vi "Agilent VNA Measure.vi"(5 "Miscellaneous Parameters":T1, 7 "Agilent VNA":T5, 8 "error in (no error)":errorcluster, 9 "SP Stimulus":T2={"Use Instrument Settings"=FALSE, "Blank Frequencies"=FALSE, "Sweep Type"=enum."Linear", "Sweep"={"Fstart"=500.0, "Fstop"=1500.0, "Units"=enum."MHz", "Points"=201}, "Power (dBm)"=999.0, "IFBW (Hz)"=-1.0, "Sweep Time (s)"=-1.0, "Calibration"={"State"=FALSE, "String"=""}} {"Sweep Time (s)" format="%.3g"}, 10 "Parameters to Measure":T6[](array[typedef]) {"Channel" min=1 max=99 step=1; "Parameter"."Stimulus Port" min=1 step=1; "Parameter"."Response Port" min=1 step=1}, 11 "VISA Resource Name":refnum<visa-resource-name>) -> (0 "error out":errorcluster, 1 "S Parameters":cluster{"f0":dbl, "df":dbl, cdb[][]}, 2 "Parameters to Measure":T6[](array[typedef]) {"Channel" min=1 max=99 step=1; "Parameter"."Stimulus Port" min=1 step=1; "Parameter"."Response Port" min=1 step=1}, 3 "dup VISA Resource Name":refnum<visa-resource-name>)   [LabVIEW 2011]
uses:
  tests/S Parameter/TypeDefs/SP Parameter to Measure.ctl
  tests/S Parameter/TypeDefs/SP Parameter.ctl
  tests/S Parameter/TypeDefs/SP Calibration State.ctl
  tests/S Parameter/TypeDefs/SP Measurement Format.ctl
  TypeDefs/Agilent VNA Instrument Info.ctl
  tests/S Parameter/TypeDefs/SP Stimulus Parameters.ctl
  tests/S Parameter/TypeDefs/SP Frequency Units.ctl
  tests/S Parameter/TypeDefs/SP Miscellaneous Parameters.ctl
  TypeDefs/Agilent VNA External Trigger Mode.ctl
  TypeDefs/Agilent VNA Measurement.ctl
  TypeDefs/Agilent VNA Trigger Mode.ctl
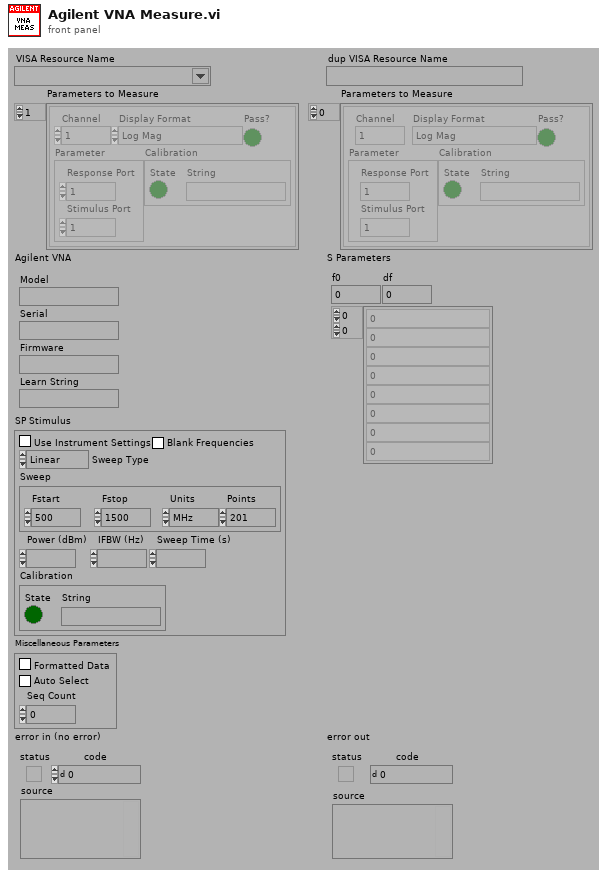
[diagram p1: front panel]
types:
  T1 = typedef "SP Miscellaneous Parameters.ctl" = cluster{"Formatted Data":bool, "Auto Select":bool, "Seq Count":u32}
  T2 = typedef "SP Stimulus Parameters.ctl" = cluster{"Use Instrument Settings":bool, "Blank Frequencies":bool, "Sweep Type":enum32{"Linear", "Logarithmic", "List", "Power", "CW"}, "Sweep":cluster{"Fstart":dbl, "Fstop":dbl, "Units":T3, "Points":i32}, "Power (dBm)":dbl, "IFBW (Hz)":dbl, "Sweep Time (s)":dbl, "Calibration":T4}
  T3 = typedef "SP Frequency Units.ctl" = enum16{"Hz", "kHz", "MHz", "GHz", "Points"}
  T4 = typedef "SP Calibration State.ctl" = cluster{"State":bool, "String":string}
  T5 = typedef "Agilent VNA Instrument Info.ctl" = cluster{"Model":string, "Serial":string, "Firmware":string, "Learn String":string}
  T6 = typedef "SP Parameter to Measure.ctl" = cluster{"Channel":i8, "Parameter":T7, "Calibration":T4, "Display Format":T8, "Pass?":bool}
  T7 = typedef "SP Parameter.ctl" = cluster{"Stimulus Port":i8, "Response Port":i8}
  T8 = typedef "SP Measurement Format.ctl" = enum32{"Log Mag", "Phase", "Delay", "Smith (R+jX)", "Polar (Re/Im)", "Linear Mag", "SWR", "Real", "Imaginary", "Smith (Lin/Phase)", "Smith (Log/Phase)", "Smith (Real/Imag)", "Smith (G+jB)", "Polar (Lin/Phase)", "Polar (Log/Phase)", "Expanded Phase", "Positive Phase", "Inverted Smith", "Unwrapped Phase", "Power Out", "Power In", "Linear Mag/Phase", "Log Mag/Phase", "Real/Imaginary"}
  T9 = typedef "Agilent VNA Model.ctl" = enum16{"Not Supported", "8510X", "8719X", "8720X", "8722X", "8753X", "ENA", "PNA", "Field Fox"}
  T10 = typedef "Agilent VNA Measurements.ctl" = cluster{"Channel":i8, "Traces":cluster{"Trace":i8, "Parameter":T7}[]}
  T11 = typedef "Agilent VNA External Trigger Mode.ctl" = enum16{"Off", "On Sweep", "On Point", "Manual On Point", "Internal", "External", "Bus"}
  T12 = typedef "Agilent VNA Measurement.ctl" = enum32{"SXX", "Analog In - Aux In", "A/R", "B/R", "A/B", "A", "B", "R"}
  T13 = typedef "Agilent VNA Trigger Mode.ctl" = enum16{"Continuous", "Hold", "Single"}
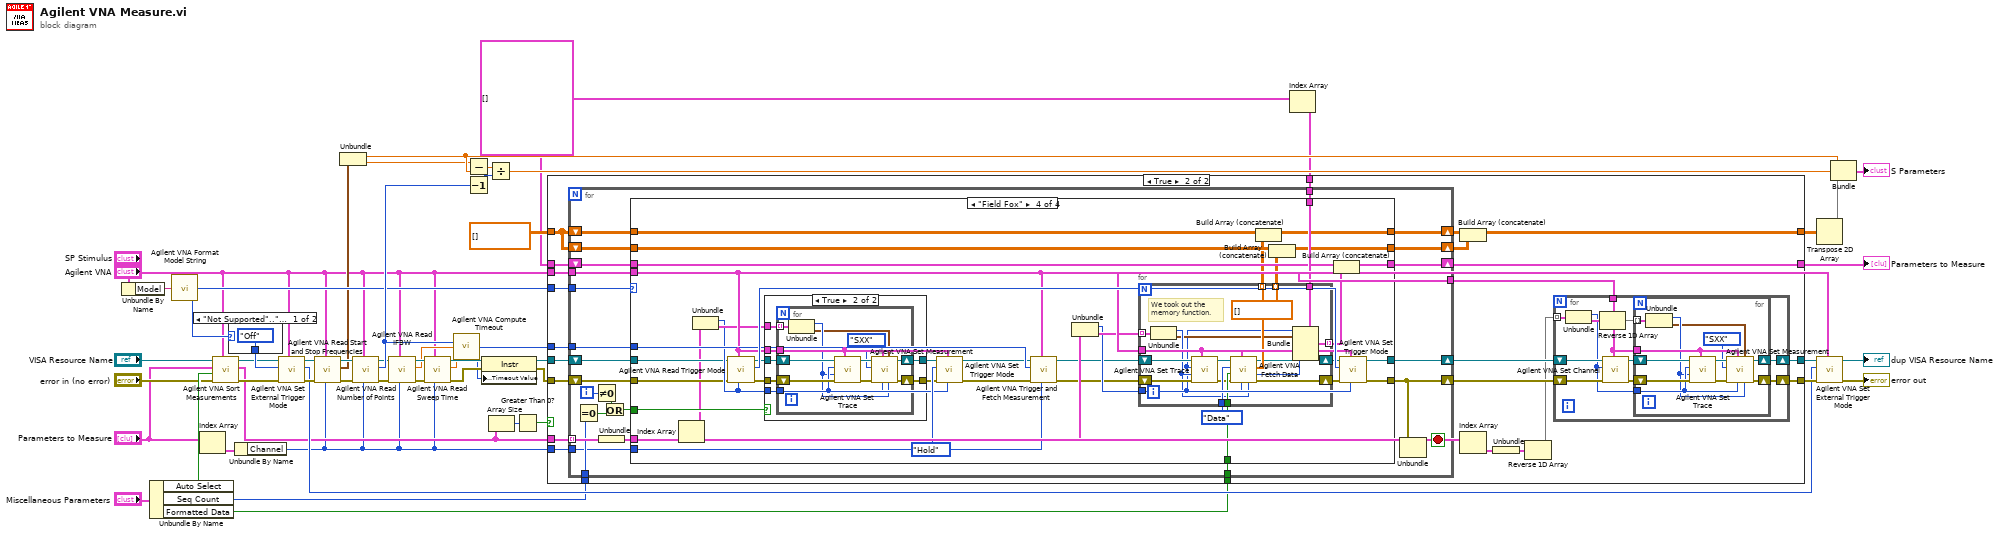
[diagram p0: block diagram]
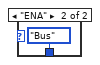
[diagram p2: hidden frame]
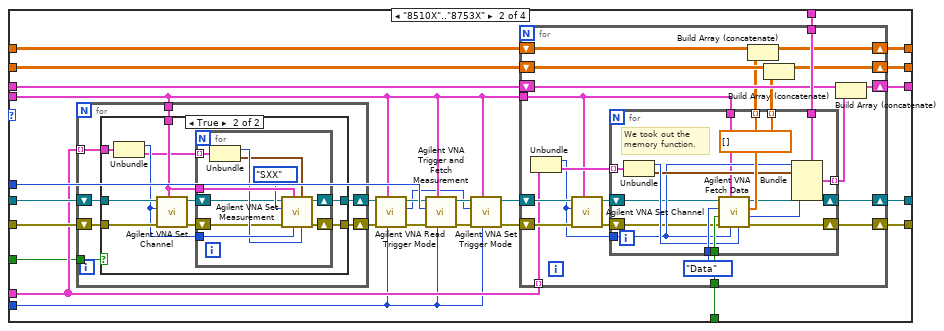
[diagram p5: hidden frame]
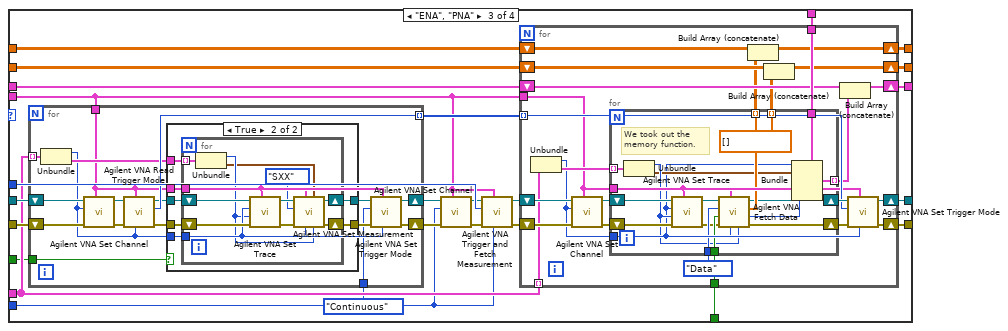
[diagram p7: hidden frame]
diagram:
  w17 = T6[] [] ("Parameters to Measure")
  n1 = Unbundle By Name("Agilent VNA") -> ("Model"=w15:string)
  n2 = Unbundle By Name("Miscellaneous Parameters") -> ("Auto Select"=w9:bool, "Seq Count"=w11:u32, "Formatted Data"=w12:bool)
  n3 = call "Agilent VNA Format Model String.vi"("Model"=w15) -> ("Model"=w14:T9)
  n4 = Index Array(array="Parameters to Measure") -> (element=w3:T6)  [unwired: 1 in]
  n5 = call "Agilent VNA Sort Measurements.vi"("Agilent VNA"="Agilent VNA", "error in (no error)"="error in (no error)", "Auto Select"=w9, "Parameters to Measure"="Parameters to Measure", "VISA Resource Name"="VISA Resource Name") -> ("error out"=w6:errorcluster, "Sorted Measurements"=w4:cluster{"Measurements":T10[]}[], "dup VISA Resource Name"=w7:refnum<visa-resource-name>)  [unwired: 4 out]
  n6 = case shown="\"Not Supported\"..\"8753X\", \"PNA\", \"Field Fox\"" w14 {
    tunnel: [Agilent_VNA_External_Trigger_Mode."Off" ("Ext. Trigger Mode") Agilent_VNA_External_Trigger_Mode."Bus" ("Ext. Trigger Mode")] -> w37
    frame "Not Supported".."8753X", "PNA", "Field Fox" {
    }
    frame "ENA" {
    }
  }
  n7 = Unbundle By Name(w3) -> ("Channel"=w1:i8)
  n8 = call "Agilent VNA Set External Trigger Mode.vi"("Agilent VNA"="Agilent VNA", "error in (no error)"=w6, "Ext. Trigger Mode"=w37, "VISA Resource Name"=w7) -> ("error out"=w26:errorcluster, "Previous Ext. Trigger Mode"=w19:T11, "dup VISA Resource Name"=w25:refnum<visa-resource-name>)  [unwired: 5 out]
  n9 = call "Agilent VNA Read Start and Stop Frequencies.vi"("Channel"=w1, "Agilent VNA"="Agilent VNA", "error in (no error)"=w26, "VISA Resource Name"=w25) -> ("error out"=w21:errorcluster, "Start/Stop Freqs, MHz"=w13:cluster{"Fstart":dbl, "Fstop":dbl}, "dup VISA Resource Name"=w20:refnum<visa-resource-name>)  [unwired: 5 out]
  n10 = Unbundle(w13) -> ("Fstart"=w43:dbl, "Fstop"=w42:dbl)
  n11 = call "Agilent VNA Read Number of Points.vi"("Channel"=w1, "Agilent VNA"="Agilent VNA", "error in (no error)"=w21, "VISA Resource Name"=w20) -> ("error out"=w23:errorcluster, "Number Points"=w27:i32, "dup VISA Resource Name"=w24:refnum<visa-resource-name>)  [unwired: 5 out]
  n12 = call "Agilent VNA Read IFBW.vi"("Channel"=w1, "Agilent VNA"="Agilent VNA", "error in (no error)"=w23, "VISA Resource Name"=w24) -> ("error out"=w35:errorcluster, "IFBW, Hz"=w32:dbl, "dup VISA Resource Name"=w36:refnum<visa-resource-name>)  [unwired: 5 out]
  n13 = call "Agilent VNA Read Sweep Time.vi"("Channel"=w1, "Agilent VNA"="Agilent VNA", "error in (no error)"=w35, "VISA Resource Name"=w36) -> ("error out"=w34:errorcluster, "Sweep Time, s"=w31:dbl, "dup VISA Resource Name"=w33:refnum<visa-resource-name>)  [unwired: 5 out]
  n14 = call "Agilent VNA Compute Timeout.vi"("Points"=w27, "IFBW (Hz)"=w32, "Sweep Time (s)"=w31) -> ("Timeout (ms)"=w28:u32)  [unwired: 1 in, 11 out]
  n15 = Subtract(x=w42, y=w43) -> (x-y=w51:dbl)
  n16 = Decrement(x=w27) -> (x-1=w50:i32)
  n17 = property class="Instr"(reference=w33, error in=w34, "General Settings:Timeout Value"=w28) -> (reference out=w44:refnum<visa-resource-name>, error out=w41:errorcluster)
  n18 = Divide(x=w51, y=w50) -> (x/y=w48:dbl)
  n19 = Array Size(array=w4) -> (size(s)=w46:i32)
  n20 = Greater Than 0?(x=w46) -> (x > 0?=w45:bool)
  n21 = Index Array(array=w17) -> (element=w16:T6)  [unwired: 1 in]
  n22 = case shown="True" w45 {
    tunnel: [w58 w79] -> w39
    tunnel: w44 -> [w56 w60]
    tunnel: w4 -> [_ w62]
    tunnel: [w57 w71] -> w52
    tunnel: "Agilent VNA" -> [_ w67]
    tunnel: w41 -> [w58 w59]
    tunnel: cdb[][] [] -> [w57 w74]
    tunnel: [w56 w78] -> w38
    tunnel: w28 -> [_ w75]
    tunnel: w12 -> [_ w70]
    tunnel: [w55 w69] -> w22
    tunnel: w17 -> [w55 w68]
    tunnel: w16 -> [_ w66]
    tunnel: w14 -> [_ w64]
    tunnel: w11 -> [_ w63]
    tunnel: w1 -> [_ w61]
    frame False {
    }
    frame True {
      n23 = for {
        shift-right: [w103] -> w80
        shift-left: w59 -> [w105]
        tunnel: w62 -> [w90] mode=indexing
        tunnel: w67 -> [w92]
        shift-right: [w93] -> w72
        shift-left: w74 -> [w98]
        shift-right: [w104] -> w81
        shift-left: w60 -> [w106]
        tunnel: [w92] -> w76
        tunnel: w75 -> [w102]
        shift-right: [w94] -> w73
        shift-left: w74 -> [w97]
        tunnel: w70 -> [w101]
        shift-right: [w95] -> w69
        shift-left: w68 -> [w96]
        tunnel: w66 -> [w99]
        tunnel: w64 -> [w91]
        tunnel: w63 -> [w85]
        tunnel: w61 -> [w83]
        i -> [w86]
        stop <- w100 stop-if-true
        n24 = Equal To 0?(x=w85) -> (x = 0?=w88:bool)
        n25 = Not Equal To 0?(x=w86) -> (x != 0?=w87:bool)
        n26 = Unbundle(w90) -> ("Measurements"=w89:T10[])
        n27 = Or(x=w87, y=w88) -> (x .or. y?=w84:bool)
        n28 = case shown="\"Field Fox\"" w91 {
          tunnel: w106 -> [w110 w137 w229 w324]
          tunnel: w105 -> [w111 w136 w228 w325]
          tunnel: [w110 w135 w223 w348] -> w104
          tunnel: [w111 w134 w222 w347] -> w103
          tunnel: w102 -> [_ w133 w220 w345]
          tunnel: w101 -> [_ w132 w219 w344]
          tunnel: w99 -> [_ w131 w218 w343]
          tunnel: w98 -> [w108 w130 w217 w342]
          tunnel: w97 -> [w109 w129 w216 w341]
          tunnel: w96 -> [w107 w128 w215 w340]
          tunnel: [w107 w127 w214 w339] -> w95
          tunnel: [w109 w126 w213 w338] -> w94
          tunnel: [w108 w125 w212 w337] -> w93
          tunnel: w92 -> [_ w115 w211 w336]
          tunnel: w89 -> [_ w124 w208 w332]
          tunnel: w84 -> [_ w113 w207 w335]
          tunnel: w83 -> [_ w112 w205 w333]
          frame "Not Supported" {
          }
          frame "8510X".."8753X" {
            n29 = for {
              tunnel: w115 -> [w177]
              tunnel: w124 -> [w180] mode=indexing
              shift-right: [w178] -> w122
              shift-left: w136 -> [w181]
              shift-right: [w179] -> w123
              shift-left: w137 -> [w182]
              tunnel: w113 -> [w176]
              n30 = case shown="True" w176 {
                tunnel: w182 -> [w184 w194]
                tunnel: w181 -> [w183 w193]
                tunnel: w180 -> [_ w192]
                tunnel: [w184 w191] -> w179
                tunnel: [w183 w190] -> w178
                tunnel: w177 -> [_ w189]
                frame False {
                  # "Save time because we know that the previous\nrun set these measurements back to the first\nparameters.  The cannot be skipped if it is the\nsecond measurement in a run though or if it is\nthe first time through."
                }
                frame True {
                  n31 = Unbundle(w192) -> ("Channel"=w188:i8, "Traces"=w187:cluster{"Trace":i8, "Parameter":T7}[])
                  n32 = call "Agilent VNA Set Channel.vi"("Agilent VNA"=w189, "error in (no error)"=w193, "Channel"=w188, "VISA Resource Name"=w194) -> ("error out"=w186:errorcluster, "dup VISA Resource Name"=w185:refnum<visa-resource-name>)  [unwired: 6 out]
                  n33 = for {
                    tunnel: w189 -> [w202]
                    tunnel: w188 -> [w201]
                    tunnel: w187 -> [w200] mode=indexing
                    shift-right: [w204] -> w191
                    shift-left: w185 -> [w196]
                    shift-right: [w203] -> w190
                    shift-left: w186 -> [w195]
                    n34 = Unbundle(w200) -> ("Trace"=w199:i8, "Parameter"=w197:T7)
                    n35 = call "Agilent VNA Set Measurement.vi"("Trace"=w199, "Parameter"=w197, "Channel"=w201, "Agilent VNA"=w202, "error in (no error)"=w195, "Measurement (SXX)"=Agilent_VNA_Measurement."SXX" ("Measurement (S11 - A/R)"), "VISA Resource Name"=w196) -> ("error out"=w203:errorcluster, "dup VISA Resource Name"=w204:refnum<visa-resource-name>)  [unwired: 1 in, 2 out]
                  }
                }
              }
            }
            n36 = call "Agilent VNA Read Trigger Mode.vi"("Channel"=w112, "Agilent VNA"=w115, "error in (no error)"=w122, "VISA Resource Name"=w123) -> ("error out"=w121:errorcluster, "Trigger Mode"=w114:T13, "dup VISA Resource Name"=w120:refnum<visa-resource-name>)  [unwired: 5 out]
            n37 = call "Agilent VNA Trigger and Fetch Measurement.vi"("Channel"=w112, "Agilent VNA"=w115, "error in (no error)"=w121, "Timout, ms (10000)"=w133, "VISA Resource Name"=w120) -> ("error out"=w119:errorcluster, "dup VISA Resource Name"=w118:refnum<visa-resource-name>)  [unwired: 1 in, 4 out]
            n38 = call "Agilent VNA Set Trigger Mode.vi"("Channel"=w112, "Agilent VNA"=w115, "error in (no error)"=w119, "Trigger Mode"=w114, "VISA Resource Name"=w118) -> ("error out"=w116:errorcluster, "dup VISA Resource Name"=w117:refnum<visa-resource-name>)  [unwired: 5 out]
            n39 = for {
              shift-right: [w139] -> w134
              shift-left: w116 -> [w159]
              tunnel: w124 -> [w152] mode=indexing
              shift-right: [w140] -> w135
              shift-left: w117 -> [w158]
              tunnel: w132 -> [w156]
              tunnel: w131 -> [w153]
              tunnel: w115 -> [w138]
              shift-right: [w146] -> w125
              shift-left: w130 -> [w149]
              shift-right: [w144] -> w127
              shift-left: w128 -> [w147]
              shift-right: [w145] -> w126
              shift-left: w129 -> [w148]
              n40 = Unbundle(w152) -> ("Channel"=w150:i8, "Traces"=w151:cluster{"Trace":i8, "Parameter":T7}[])
              n41 = call "Agilent VNA Set Channel.vi"("Agilent VNA"=w138, "error in (no error)"=w159, "Channel"=w150, "VISA Resource Name"=w158) -> ("error out"=w154:errorcluster, "dup VISA Resource Name"=w155:refnum<visa-resource-name>)  [unwired: 6 out]
              n42 = for {
                tunnel: [w175] -> w141 mode=indexing
                tunnel: [cdb[] [] ("Data (real+imag)")] -> w142 mode=indexing
                tunnel: enum16{"Data", "Memory"}."Data" ("Data to Read (Data)") -> [w174]
                tunnel: w156 -> [w173]
                tunnel: [w171] -> w143 mode=indexing
                tunnel: w150 -> [w166]
                tunnel: w153 -> [w170]
                shift-right: [w164] -> w140
                shift-left: w155 -> [w162]
                shift-right: [w163] -> w139
                shift-left: w154 -> [w161]
                tunnel: w151 -> [w169] mode=indexing
                tunnel: w138 -> [w160]
                # "We took out the\nmemory function."
                n43 = Unbundle(w169) -> ("Trace"=w168:i8, "Parameter"=w167:T7)
                n44 = call "Agilent VNA Fetch Data.vi"("Trace"=w168, "Channel"=w166, "Agilent VNA"=w160, "error in (no error)"=w161, "Formatted Data?"=w173, "Data to Read (Data)"=w174, "VISA Resource Name"=w162) -> ("error out"=w163:errorcluster, "Display Format"=w172:T8, "Data (real+imag)"=w175:cdb[], "dup VISA Resource Name"=w164:refnum<visa-resource-name>)  [unwired: 1 out]
                n45 = Bundle(cluster=w170, "Channel"=w166, "Parameter"=w167, "Display Format"=w172) -> (w171:T6)  [unwired: 2 out]
              }
              n46 = Build Array (concatenate)(w149, w141) -> (w146:cdb[][])
              n47 = Build Array (concatenate)(w148, w142) -> (w145:cdb[][])
              n48 = Build Array (concatenate)(w147, w143) -> (w144:T6[])
            }
          }
          frame "ENA", "PNA" {
            n49 = for {
              tunnel: w211 -> [w276]
              tunnel: w208 -> [w287] mode=indexing
              shift-right: [w277] -> w225
              shift-left: w228 -> [w288]
              shift-right: [w279] -> w224
              shift-left: w229 -> [w289]
              tunnel: [w284] -> w221 mode=indexing
              tunnel: w207 -> [w274]
              tunnel: Agilent_VNA_Trigger_Mode."Continuous" ("Trigger Mode") -> [w273]
              n50 = Unbundle(w287) -> ("Channel"=w275:i8, "Traces"=w281:cluster{"Trace":i8, "Parameter":T7}[])
              n51 = call "Agilent VNA Set Channel.vi"("Agilent VNA"=w276, "error in (no error)"=w288, "Channel"=w275, "VISA Resource Name"=w289) -> ("error out"=w285:errorcluster, "dup VISA Resource Name"=w286:refnum<visa-resource-name>)  [unwired: 6 out]
              n52 = call "Agilent VNA Read Trigger Mode.vi"("Channel"=w275, "Agilent VNA"=w276, "error in (no error)"=w285, "VISA Resource Name"=w286) -> ("error out"=w283:errorcluster, "Trigger Mode"=w284:T13, "dup VISA Resource Name"=w282:refnum<visa-resource-name>)  [unwired: 5 out]
              n53 = case shown="True" w274 {
                tunnel: w283 -> [w290 w298]
                tunnel: w282 -> [w291 w297]
                tunnel: w281 -> [_ w296]
                tunnel: [w291 w295] -> w280
                tunnel: [w290 w294] -> w278
                tunnel: w276 -> [_ w293]
                tunnel: w275 -> [_ w292]
                frame False {
                  # "Save time because we know that the previousrun set these measurements back to the first parameters.  They cannot be skipped if it is the second measurement in a run though or if it isthe first time through."
                }
                frame True {
                  n54 = for {
                    tunnel: w293 -> [w304]
                    tunnel: w292 -> [w303]
                    tunnel: w296 -> [w302] mode=indexing
                    shift-right: [w310] -> w295
                    shift-left: w297 -> [w305]
                    shift-right: [w309] -> w294
                    shift-left: w298 -> [w308]
                    n55 = Unbundle(w302) -> ("Trace"=w301:i8, "Parameter"=w299:T7)
                    n56 = call "Agilent VNA Set Trace.vi"("Agilent VNA"=w304, "error in (no error)"=w308, "Trace"=w301, "Channel"=w303, "VISA Resource Name"=w305) -> ("error out"=w307:errorcluster, "dup VISA Resource Name"=w306:refnum<visa-resource-name>)  [unwired: 5 out]
                    n57 = call "Agilent VNA Set Measurement.vi"("Trace"=w301, "Parameter"=w299, "Channel"=w303, "Agilent VNA"=w304, "error in (no error)"=w307, "Measurement (SXX)"=Agilent_VNA_Measurement."SXX" ("Measurement (S11 - A/R)"), "VISA Resource Name"=w306) -> ("error out"=w309:errorcluster, "dup VISA Resource Name"=w310:refnum<visa-resource-name>)  [unwired: 1 in, 2 out]
                  }
                }
              }
              n58 = call "Agilent VNA Set Trigger Mode.vi"("Channel"=w275, "Agilent VNA"=w276, "error in (no error)"=w278, "Trigger Mode"=w273, "VISA Resource Name"=w280) -> ("error out"=w277:errorcluster, "dup VISA Resource Name"=w279:refnum<visa-resource-name>)  [unwired: 5 out]
            }
            n59 = call "Agilent VNA Set Channel.vi"("Agilent VNA"=w211, "error in (no error)"=w225, "Channel"=w205, "VISA Resource Name"=w224) -> ("error out"=w210:errorcluster, "dup VISA Resource Name"=w209:refnum<visa-resource-name>)  [unwired: 6 out]
            n60 = call "Agilent VNA Trigger and Fetch Measurement.vi"("Channel"=w205, "Agilent VNA"=w211, "error in (no error)"=w210, "Timout, ms (10000)"=w220, "VISA Resource Name"=w209) -> ("error out"=w227:errorcluster, "dup VISA Resource Name"=w226:refnum<visa-resource-name>)  [unwired: 1 in, 4 out]
            n61 = for {
              shift-right: [w242] -> w222
              shift-left: w227 -> [w254]
              tunnel: w208 -> [w247] mode=indexing
              shift-right: [w244] -> w223
              shift-left: w226 -> [w253]
              tunnel: w221 -> [w240] mode=indexing
              tunnel: w219 -> [w251]
              tunnel: w218 -> [w248]
              tunnel: w211 -> [w239]
              shift-right: [w235] -> w212
              shift-left: w217 -> [w238]
              shift-right: [w233] -> w214
              shift-left: w215 -> [w236]
              shift-right: [w234] -> w213
              shift-left: w216 -> [w237]
              n62 = Unbundle(w247) -> ("Channel"=w241:i8, "Traces"=w246:cluster{"Trace":i8, "Parameter":T7}[])
              n63 = call "Agilent VNA Set Channel.vi"("Agilent VNA"=w239, "error in (no error)"=w254, "Channel"=w241, "VISA Resource Name"=w253) -> ("error out"=w249:errorcluster, "dup VISA Resource Name"=w250:refnum<visa-resource-name>)  [unwired: 6 out]
              n64 = for {
                tunnel: [w272] -> w230 mode=indexing
                tunnel: [cdb[] [] ("Data (real+imag)")] -> w231 mode=indexing
                tunnel: enum16{"Data", "Memory"}."Data" ("Data to Read (Data)") -> [w271]
                tunnel: w251 -> [w270]
                tunnel: [w268] -> w232 mode=indexing
                tunnel: w239 -> [w263]
                tunnel: w241 -> [w258]
                tunnel: w248 -> [w262]
                shift-right: [w256] -> w245
                shift-left: w250 -> [w267]
                shift-right: [w255] -> w243
                shift-left: w249 -> [w266]
                tunnel: w246 -> [w261] mode=indexing
                # "We took out the\nmemory function."
                n65 = Unbundle(w261) -> ("Trace"=w260:i8, "Parameter"=w259:T7)
                n66 = call "Agilent VNA Set Trace.vi"("Agilent VNA"=w263, "error in (no error)"=w266, "Trace"=w260, "Channel"=w258, "VISA Resource Name"=w267) -> ("error out"=w265:errorcluster, "dup VISA Resource Name"=w264:refnum<visa-resource-name>)  [unwired: 5 out]
                n67 = call "Agilent VNA Fetch Data.vi"("Trace"=w260, "Channel"=w258, "Agilent VNA"=w263, "error in (no error)"=w265, "Formatted Data?"=w270, "Data to Read (Data)"=w271, "VISA Resource Name"=w264) -> ("error out"=w255:errorcluster, "Display Format"=w269:T8, "Data (real+imag)"=w272:cdb[], "dup VISA Resource Name"=w256:refnum<visa-resource-name>)  [unwired: 1 out]
                n68 = Bundle(cluster=w262, "Channel"=w258, "Parameter"=w259, "Display Format"=w269) -> (w268:T6)  [unwired: 2 out]
              }
              n69 = Build Array (concatenate)(w238, w230) -> (w235:cdb[][])
              n70 = Build Array (concatenate)(w237, w231) -> (w234:cdb[][])
              n71 = Build Array (concatenate)(w236, w232) -> (w233:T6[])
              n72 = call "Agilent VNA Set Trigger Mode.vi"("Channel"=w241, "Agilent VNA"=w239, "error in (no error)"=w243, "Trigger Mode"=w240, "VISA Resource Name"=w245) -> ("error out"=w242:errorcluster, "dup VISA Resource Name"=w244:refnum<visa-resource-name>)  [unwired: 5 out]
            }
          }
          frame "Field Fox" {
            n73 = Index Array(array=w332) -> (element=w313:T10)  [unwired: 1 in]
            n74 = Unbundle(w313) -> ("Channel"=w326:i8, "Traces"=w329:cluster{"Trace":i8, "Parameter":T7}[])
            n75 = call "Agilent VNA Read Trigger Mode.vi"("Channel"=w326, "Agilent VNA"=w336, "error in (no error)"=w325, "VISA Resource Name"=w324) -> ("error out"=w331:errorcluster, "Trigger Mode"=w346:T13, "dup VISA Resource Name"=w330:refnum<visa-resource-name>)  [unwired: 5 out]
            n76 = case shown="True" w335 {
              tunnel: w331 -> [w367 w375]
              tunnel: w330 -> [w368 w374]
              tunnel: w329 -> [_ w373]
              tunnel: [w368 w372] -> w328
              tunnel: [w367 w371] -> w327
              tunnel: w336 -> [_ w370]
              tunnel: w326 -> [_ w369]
              frame False {
                # "Save time because we know that the previousrun set these measurements back to the first parameters.  They cannot be skipped if it is the second measurement in a run though or if it isthe first time through."
              }
              frame True {
                n77 = for {
                  tunnel: w370 -> [w381]
                  tunnel: w369 -> [w380]
                  tunnel: w373 -> [w379] mode=indexing
                  shift-right: [w387] -> w372
                  shift-left: w374 -> [w382]
                  shift-right: [w386] -> w371
                  shift-left: w375 -> [w385]
                  n78 = Unbundle(w379) -> ("Trace"=w378:i8, "Parameter"=w376:T7)
                  n79 = call "Agilent VNA Set Trace.vi"("Agilent VNA"=w381, "error in (no error)"=w385, "Trace"=w378, "Channel"=w380, "VISA Resource Name"=w382) -> ("error out"=w384:errorcluster, "dup VISA Resource Name"=w383:refnum<visa-resource-name>)  [unwired: 5 out]
                  n80 = call "Agilent VNA Set Measurement.vi"("Trace"=w378, "Parameter"=w376, "Channel"=w380, "Agilent VNA"=w381, "error in (no error)"=w384, "Measurement (SXX)"=Agilent_VNA_Measurement."SXX" ("Measurement (S11 - A/R)"), "VISA Resource Name"=w383) -> ("error out"=w386:errorcluster, "dup VISA Resource Name"=w387:refnum<visa-resource-name>)  [unwired: 1 in, 2 out]
                }
              }
            }
            n81 = call "Agilent VNA Set Trigger Mode.vi"("Channel"=w326, "Agilent VNA"=w336, "error in (no error)"=w327, "Trigger Mode"=Agilent_VNA_Trigger_Mode."Hold", "VISA Resource Name"=w328) -> ("error out"=w322:errorcluster, "dup VISA Resource Name"=w323:refnum<visa-resource-name>)  [unwired: 5 out]
            n82 = call "Agilent VNA Trigger and Fetch Measurement.vi"("Channel"=w333, "Agilent VNA"=w336, "error in (no error)"=w322, "Timout, ms (10000)"=w345, "VISA Resource Name"=w323) -> ("error out"=w311:errorcluster, "dup VISA Resource Name"=w312:refnum<visa-resource-name>)  [unwired: 1 in, 4 out]
            n83 = Unbundle(w313) -> ("Channel"=w317:i8, "Traces"=w320:cluster{"Trace":i8, "Parameter":T7}[])
            n84 = for {
              tunnel: [w366] -> w314 mode=indexing
              tunnel: [cdb[] [] ("Data (real+imag)")] -> w315 mode=indexing
              tunnel: enum16{"Data", "Memory"}."Data" ("Data to Read (Data)") -> [w365]
              tunnel: w344 -> [w364]
              tunnel: [w362] -> w316 mode=indexing
              tunnel: w336 -> [w357]
              tunnel: w317 -> [w352]
              tunnel: w343 -> [w356]
              shift-right: [w350] -> w319
              shift-left: w312 -> [w361]
              shift-right: [w349] -> w318
              shift-left: w311 -> [w360]
              tunnel: w320 -> [w355] mode=indexing
              # "We took out the\nmemory function."
              n85 = Unbundle(w355) -> ("Trace"=w354:i8, "Parameter"=w353:T7)
              n86 = call "Agilent VNA Set Trace.vi"("Agilent VNA"=w357, "error in (no error)"=w360, "Trace"=w354, "Channel"=w352, "VISA Resource Name"=w361) -> ("error out"=w359:errorcluster, "dup VISA Resource Name"=w358:refnum<visa-resource-name>)  [unwired: 5 out]
              n87 = call "Agilent VNA Fetch Data.vi"("Trace"=w354, "Channel"=w352, "Agilent VNA"=w357, "error in (no error)"=w359, "Formatted Data?"=w364, "Data to Read (Data)"=w365, "VISA Resource Name"=w358) -> ("error out"=w349:errorcluster, "Display Format"=w363:T8, "Data (real+imag)"=w366:cdb[], "dup VISA Resource Name"=w350:refnum<visa-resource-name>)  [unwired: 1 out]
              n88 = Bundle(cluster=w356, "Channel"=w352, "Parameter"=w353, "Display Format"=w363) -> (w362:T6)  [unwired: 2 out]
            }
            n89 = Build Array (concatenate)(w342, w314) -> (w337:cdb[][])
            n90 = Build Array (concatenate)(w341, w315) -> (w338:cdb[][])
            n91 = Build Array (concatenate)(w340, w316) -> (w339:T6[])
            n92 = call "Agilent VNA Set Trigger Mode.vi"("Channel"=w317, "Agilent VNA"=w336, "error in (no error)"=w318, "Trigger Mode"=w346, "VISA Resource Name"=w319) -> ("error out"=w347:errorcluster, "dup VISA Resource Name"=w348:refnum<visa-resource-name>)  [unwired: 5 out]
          }
        }
        n93 = Unbundle(w103) -> ("status"=w100:bool)  [unwired: 2 out]
      }
      n94 = Build Array (concatenate)(w72, w73) -> (w71:cdb[][])
      n95 = Index Array(array=w62) -> (element=w82:cluster{"Measurements":T10[]})  [unwired: 1 in]
      n96 = Unbundle(w82) -> ("Measurements"=w65:T10[])
      n97 = Reverse 1D Array(array=w65) -> (reversed array=w77:T10[])
      n98 = for {
        tunnel: w76 -> [w393]
        tunnel: w77 -> [w396] mode=indexing
        shift-right: [w390] -> w79
        shift-left: w80 -> [w397]
        shift-right: [w389] -> w78
        shift-left: w81 -> [w398]
        n99 = Unbundle(w396) -> ("Channel"=w391:i8, "Traces"=w392:cluster{"Trace":i8, "Parameter":T7}[])
        n100 = Reverse 1D Array(array=w392) -> (reversed array=w388:cluster{"Trace":i8, "Parameter":T7}[])
        n101 = call "Agilent VNA Set Channel.vi"("Agilent VNA"=w393, "error in (no error)"=w397, "Channel"=w391, "VISA Resource Name"=w398) -> ("error out"=w395:errorcluster, "dup VISA Resource Name"=w394:refnum<visa-resource-name>)  [unwired: 6 out]
        n102 = for {
          tunnel: w393 -> [w404]
          tunnel: w391 -> [w403]
          tunnel: w388 -> [w402] mode=indexing
          shift-right: [w410] -> w389
          shift-left: w394 -> [w405]
          shift-right: [w409] -> w390
          shift-left: w395 -> [w408]
          n103 = Unbundle(w402) -> ("Trace"=w401:i8, "Parameter"=w400:T7)
          n104 = call "Agilent VNA Set Trace.vi"("Agilent VNA"=w404, "error in (no error)"=w408, "Trace"=w401, "Channel"=w403, "VISA Resource Name"=w405) -> ("error out"=w407:errorcluster, "dup VISA Resource Name"=w406:refnum<visa-resource-name>)  [unwired: 5 out]
          n105 = call "Agilent VNA Set Measurement.vi"("Trace"=w401, "Parameter"=w400, "Channel"=w403, "Agilent VNA"=w404, "error in (no error)"=w407, "Measurement (SXX)"=Agilent_VNA_Measurement."SXX" ("Measurement (S11 - A/R)"), "VISA Resource Name"=w406) -> ("error out"=w409:errorcluster, "dup VISA Resource Name"=w410:refnum<visa-resource-name>)  [unwired: 1 in, 2 out]
        }
      }
    }
  }
  "Parameters to Measure" <- w22
  n106 = Transpose 2D Array(2D array=w52) -> (transposed array=w47:cdb[][])
  n107 = call "Agilent VNA Set External Trigger Mode.vi"("Agilent VNA"="Agilent VNA", "error in (no error)"=w39, "Ext. Trigger Mode"=w19, "VISA Resource Name"=w38) -> ("error out"=→"error out":errorcluster, "dup VISA Resource Name"=→"dup VISA Resource Name":refnum<visa-resource-name>)  [unwired: 6 out]
  n108 = Bundle("Fstart"=w43, w48, w47) -> (→"S Parameters":cluster{"Fstart":dbl, dbl, cdb[][]})  [unwired: 1 out]
